vi "Stack.vi"(8 "error in":errorcluster, 10 "RC?":bool, 11 "Teir":T1) -> ()   [LabVIEW 2014, in "Elevator System.lvlib"]
uses:
  Elevator System.lvlib
  Typedef/TeirNumber.ctl
  Typedef/MessageType.ctl
  Typedef/Commands.ctl
  Typedef/StackMessage.ctl
  Typedef/StackCommandType.ctl
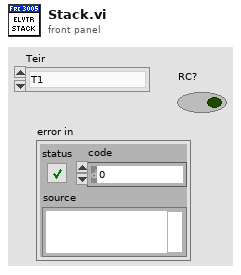
[diagram p1: front panel]
types:
  T1 = typedef "Elevator System.lvlib/TeirNumber.ctl" = enum16{"T1", "T2", "T3", "T4", "T5", "T6"}
  T2 = typedef "Elevator System.lvlib/StackCommandType.ctl" = enum16{"Normal", "RC", "Step"}
  T3 = typedef "Elevator System.lvlib/StackMessage.ctl" = cluster{"Type":T2, "Teir":T1}
  T4 = typedef "Elevator System.lvlib/Commands.ctl" = enum16{"Home", "Stack", "Pickup", "Score", "Cycle", "Stop", "Manual Open", "Manual Close", "Manual Up", "Manual Down", "Gripper RC", "Gripper Cycle", "Wait On Gripper", "Wait On Elevator"}
  T5 = typedef "Elevator System.lvlib/MessageType.ctl" = cluster{"Name":T4, "Data":variant}
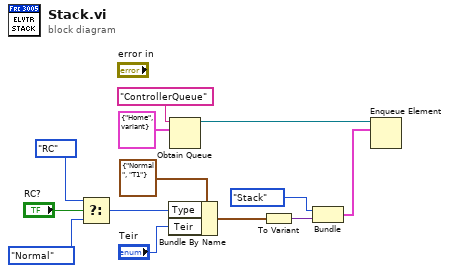
[diagram p0: block diagram]
diagram:
  n1 = Select(t=StackCommandType."RC" ("Type"), s="RC?", f=StackCommandType."Normal" ("Type")) -> (s? t:f=w2:T2)
  n2 = Bundle By Name(cluster=T3 {"Type"=enum."Normal", "Teir"=enum."T1"}, "Type"=w2, "Teir"="Teir") -> (w6:T3)
  n3 = Obtain Queue(name (unnamed)="ControllerQueue", element data type=T5 {"Name"=enum."Home", "Data"=variant} ("Message")) -> (queue out=w13:refnum<queue>)  [unwired: 3 in, 2 out]
  n4 = To Variant(anything=w6) -> (Variant=w12:variant)
  n5 = Bundle("Name"=Commands."Stack", "Variant"=w12) -> (w10:cluster{"Name":T4, "Variant":variant})  [unwired: 1 in]
  n6 = Enqueue Element(queue=w13, element=w10) -> ()  [unwired: 2 in, 3 out]
